vi "XNET Interface Property Node.vi"   [LabVIEW 2018]
doc: "Property node used to read/write properties for an XNET Interface I/O name."
uses:
  <resource>/objmgr/xnet.rc
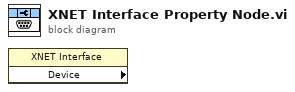
[diagram p0: block diagram]
diagram:
  n1 = property class="XNET Interface" props=["Device"]() -> ()  [unwired: 2 in, 3 out]
